vi "Get Transfer Configuration.vi"(8 "error in (no error)":errorcluster, 11 "Component Configuration in":refnum<class "Core Component Configurations.lvclass">) -> (0 "error out":errorcluster, 1 "Tx Transfer Configuration":refnum<class "Configuration.lvclass">, 2 "Rx Transfer Configuration":refnum<class "Configuration.lvclass">, 3 "Component Configuration out":refnum<class "Core Component Configurations.lvclass">)   [LabVIEW 2020, in "DSF Core.lvlib" / "Core Component Configurations.lvclass"]
uses:
  Core Component Configurations.lvclass
  Configuration/Configuration.lvclass
  Configuration/Core/Transfer/Transfer Configuration.lvclass
  C:/Users/nitest/Desktop/Git/niveristand-data-sharing-framework-custom-device/Source/Core/Classes/Configuration/Configuration.lvclass
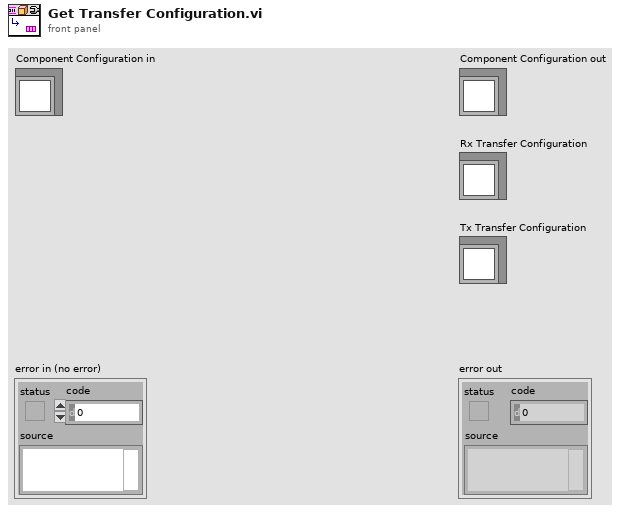
[diagram p1: front panel]
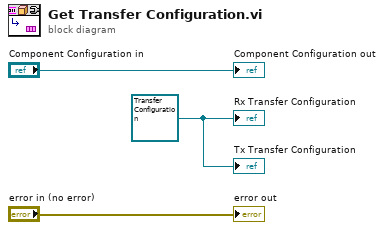
[diagram p0: block diagram]
diagram:
  w1 = refnum<class "Transfer Configuration.lvclass"> refnum ("DSF Core.lvlib:Transfer Configuration.lvclass")
  "error out" <- "error in (no error)"
  "Component Configuration out" <- "Component Configuration in"
  "Rx Transfer Configuration" <- w1
  "Tx Transfer Configuration" <- w1
